vi "Strip Comments.vi"(11 "File In":string) -> (3 "File Without Comments":string)   [LabVIEW 2019, in "LSS.lvlib"]
doc: "Removes comment sections from a style sheet text input. Comments can be in the following formats:\n\n//Single Line Comments Terminated by a Line Feed\n/*\nMulti Line Comments */\n\n<b>Inputs:</b>\n<b>File In</b> - Text from a style sheet input, still with any comments the user may have entered.\n\n<b>Outputs:</b>\n<b>File Without Comments</b> - Style sheet text with comment sections removed."
uses:
  LSS.lvlib
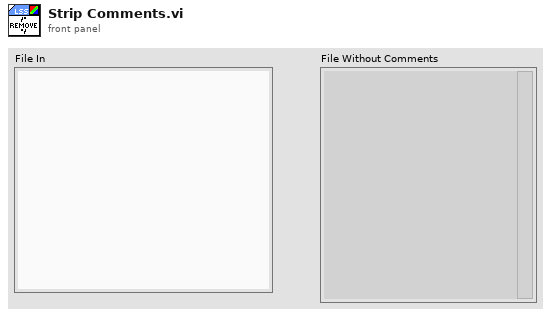
[diagram p1: front panel]
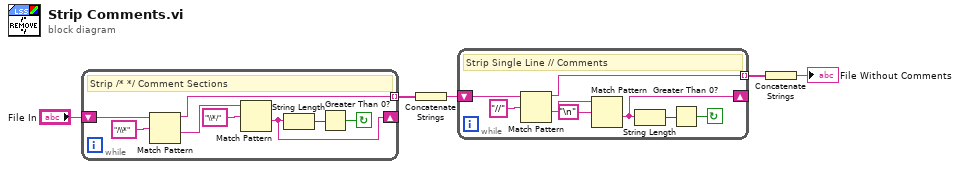
[diagram p0: block diagram]
diagram:
  n1 = while {
    tunnel: [w7] -> w5 mode=indexing
    shift-right: [w6] -> _
    shift-left: "File In" -> [w13]
    stop <- w8 continue-if-true
    # "Strip /* */ Comment Sections"
    n2 = Match Pattern(string=w13, regular expression="/\\*") -> (before substring=w7:string, after substring=w11:string)  [unwired: 1 in, 2 out]
    n3 = Match Pattern(string=w11, regular expression="\\*/") -> (after substring=w6:string)  [unwired: 1 in, 3 out]
    n4 = String Length(string=w6) -> (length=w9:i32)
    n5 = Greater Than 0?(x=w9) -> (x > 0?=w8:bool)
  }
  n6 = Concatenate Strings(w5) -> (w3:string)
  n7 = while {
    tunnel: [w16] -> w2 mode=indexing
    shift-right: [w15] -> _
    shift-left: w3 -> [w21]
    stop <- w17 continue-if-true
    # "Strip Single Line // Comments"
    n8 = Match Pattern(string=w21, regular expression="//") -> (before substring=w16:string, after substring=w19:string)  [unwired: 1 in, 2 out]
    n9 = Match Pattern(string=w19, regular expression="\n") -> (after substring=w15:string)  [unwired: 1 in, 3 out]
    n10 = String Length(string=w15) -> (length=w18:i32)
    n11 = Greater Than 0?(x=w18) -> (x > 0?=w17:bool)
  }
  n12 = Concatenate Strings(w2) -> (→"File Without Comments":string)
